vi "M14 Turret_Hardware_Begin.vi"   [LabVIEW 2019]
uses:
  <vilib>/Rock Robotics/WPI/ThirdParty/REV Robotics/SPARK MAX/Typedef/Spark MAX Idle Mode.ctl
  M14 Turret_Hardware_Globals.vi
types:
  T1 = typedef "Spark MAX Idle Mode.ctl" = enum16{"Coast", "Brake"}
  T2 = typedef "WPI_MotorControlDeviceRef.ctl" = cluster{"DeviceStatus":errorcluster, "Type":T3, "PWM":cluster{"PWM Channel":T4, "DeadBand":T5}, "CAN":cluster{"Device Number":u8, "SetOutput VI Ref":variant, "GetOutput VI Ref":variant, "Enable VI Ref":variant, "Disable VI Ref":variant, "Data":variant}, "Invert":bool, "DIO PWM":cluster{"PWM \"Enable\" Channel":T4, "DIOChannel":T6, "PWM Rate":dbl}}
  T3 = typedef "WPI_MotorControlType.ctl" = enum16{"PWM", "CAN", "DIO PWM"}
  T4 = typedef "FPGA_DIOPWMChannel.ctl" = enum8{"PWM 0", "PWM 1", "PWM 2", "PWM 3", "PWM 4", "PWM 5", "PWM 6", "PWM 7", "PWM 8", "PWM 9", "PWM MXP 0", "PWM MXP 1", "PWM MXP 2", "PWM MXP 3", "PWM MXP 4", "PWM MXP 5", "PWM MXP 6", "PWM MXP 7", "PWM MXP 8", "PWM MXP 9", "Invalid"}
  T5 = typedef "WPI_PWMDeadband.ctl" = cluster{"Name":string, "maxPositivePwm":i32, "minPositivePwm":i32, "centerPwm":i32, "maxNegativePwm":i32, "minNegativePwm":i32, "angularRange":u16}
  T6 = typedef "FPGA_DIOChannel.ctl" = enum8{"DIO 0", "DIO 1", "DIO 2", "DIO 3", "DIO 4", "DIO 5", "DIO 6", "DIO 7", "DIO 8", "DIO 9", "DIO MXP 0", "DIO MXP 1", "DIO MXP 2", "DIO MXP 3", "DIO MXP 4", "DIO MXP 5", "DIO MXP 6", "DIO MXP 7", "DIO MXP 8", "DIO MXP 9", "DIO MXP 10", "DIO MXP 11", "DIO MXP 12", "DIO MXP 13", "DIO MXP 14", "DIO MXP 15", "SPI Port CS1", "SPI Port CS2", "SPI Port CS3", "SPI Port MISO", "SPI Port MOSI", "Invalid"}
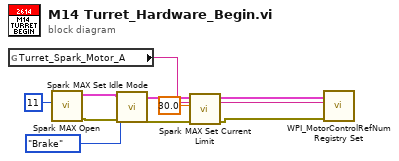
[diagram p0: block diagram]
diagram:
  n1 = global read "M14 Turret_Hardware_Globals.vi" "Turret_Spark_Motor_A"() -> (w7:string)
  n2 = call <vilib>:"Spark MAX Open.vi"("Device Number"=u8 11) -> ("error out"=w6:errorcluster, "MotorControlDeviceRef"=w9:T2)  [unwired: 9 in]
  n3 = call <vilib>:"Spark MAX Set Idle Mode.vi"("error in (no error)"=w6, "Idle Mode"=Spark_MAX_Idle_Mode."Brake", "MotorControlDeviceRef in"=w9) -> ("error out"=w4:errorcluster, "MotorControlDeviceRef out"=w5:T2)  [unwired: 7 in]
  n4 = call <vilib>:"Spark MAX Set Current Limit.vi"("error in (no error)"=w4, "Current Limit A (100)"=sgl 30.0, "MotorControlDeviceRef in"=w5) -> ("error out"=w2:errorcluster, "MotorControlDeviceRef out"=w3:T2)  [unwired: 7 in]
  n5 = call <vilib>:"WPI_MotorControlRefNum Registry Set.vi"("error in (no error)"=w2, "refnum name"=w7, "MotorControlDevRef"=w3) -> ()  [unwired: 7 in, 2 out]
